vi "VMI_radial_distri.vi"(1 "VMI in":u8[][](array[numeric]), 3 "X centre":dbl, 4 "Y centre":dbl, 5 "Radial IN":i32[](array[numeric])) -> (2 "Radial out":i32[](array[numeric]))   [LabVIEW 2015]
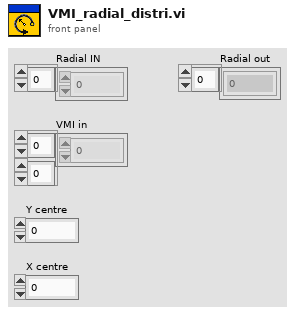
[diagram p1: front panel]
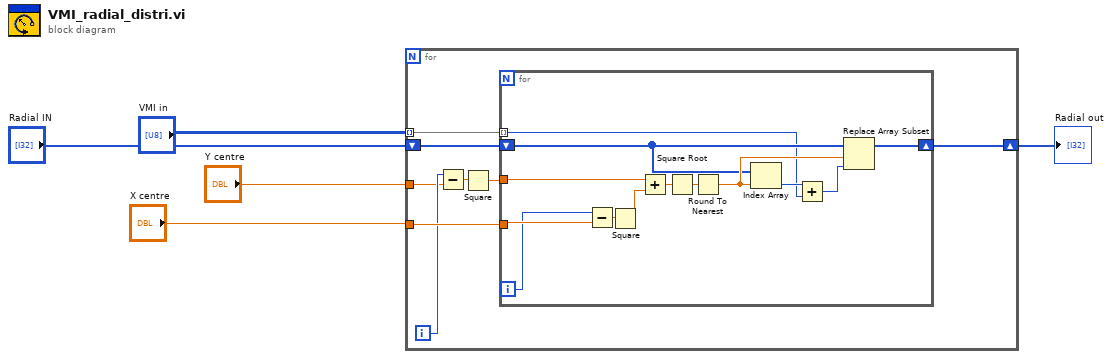
[diagram p0: block diagram]
diagram:
  n1 = for {
    tunnel: "VMI in" -> [w13] mode=indexing
    tunnel: "X centre" -> [w12]
    tunnel: "Y centre" -> [w9]
    shift-right: [w7] -> w4
    shift-left: "Radial IN" -> [w6]
    i -> [w10]
    n2 = Subtract(x=w10, y=w9) -> (x-y=w11:dbl)
    n3 = Square(x=w11) -> (x^2=w8:dbl)
    n4 = for {
      tunnel: w13 -> [w15] mode=indexing
      tunnel: w8 -> [w23]
      tunnel: w12 -> [w26]
      shift-right: [w19] -> w7
      shift-left: w6 -> [w18]
      i -> [w25]
      n5 = Subtract(x=w25, y=w26) -> (x-y=w17:dbl)
      n6 = Square(x=w17) -> (x^2=w24:dbl)
      n7 = Add(x=w23, y=w24) -> (x+y=w22:dbl)
      n8 = Square Root(x=w22) -> (sqrt(x)=w21:dbl)
      n9 = Round To Nearest(number=w21) -> (nearest integer value=w20:dbl)
      n10 = Index Array(array=w18, index=w20) -> (element=w16:i32)
      n11 = Add(x=w16, y=w15) -> (x+y=w14:i32)
      n12 = Replace Array Subset(array=w18, new element=w14, index=w20) -> (w19:i32[])
    }
  }
  "Radial out" <- w4
